vi "Periodic Tasks.vi"(8 "error in":errorcluster) -> ()   [LabVIEW 2020]
doc: "This VI runs in parallel to other tasks. It can contain as many user-defined periodic loops as you need. These can carry out PID or other sorts of timed response."
uses:
  <vilib>/Rock Robotics/WPI/Solenoid/WPI_SolenoidValue.ctl
  <vilib>/Rock Robotics/WPI/Utilities/WPI_GetSetVariantRefNum.vi
  <vilib>/Rock Robotics/Network Tables/NT Write Boolean.vi
  <vilib>/functionblocks/Edge Detection/One Shot Rising with Input/One Shot Rising with Input.vi
  <vilib>/Rock Robotics/Network Tables/NT Write Number.vi
  <vilib>/functionblocks/FB Core/FB Core.xnode
  <vilib>/Rock Robotics/WPI/Solenoid/WPI_SolenoidSetEnum.vi
  <vilib>/functionblocks/NI_FunctionBlock Libraries.lvlib
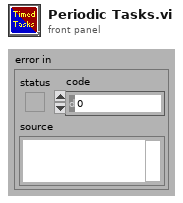
[diagram p1: front panel]
types:
  T1 = enum16{"Wait", "2 Ball", "Button Extend", "Button Retract"}
  T2 = typedef "WPI_JoystickDevRef.ctl" = cluster{"Device":T3}
  T3 = typedef "WPI_JoystickDeviceEnum.ctl" = enum16{"USB 0", "USB 1", "USB 2", "USB 3", "USB 4", "USB 5"}
  T4 = typedef "WPI_RobotDriveDevRef.ctl" = cluster{"DevStatus":errorcluster, "Motors[]":T5[], "Square Inputs":bool, "Max Output":dbl}
  T5 = typedef "WPI_MotorControlDeviceRef.ctl" = cluster{"DeviceStatus":errorcluster, "Type":T6, "PWM":cluster{"PWM Channel":T7, "DeadBand":T8}, "CAN":cluster{"Device Number":u8, "SetOutput VI Ref":variant, "GetOutput VI Ref":variant, "Enable VI Ref":variant, "Disable VI Ref":variant, "Data":variant}, "Invert":bool, "DIO PWM":cluster{"PWM \"Enable\" Channel":T7, "DIOChannel":T9, "PWM Rate":dbl}}
  T6 = typedef "WPI_MotorControlType.ctl" = enum16{"PWM", "CAN", "DIO PWM"}
  T7 = typedef "FPGA_DIOPWMChannel.ctl" = enum8{"PWM 0", "PWM 1", "PWM 2", "PWM 3", "PWM 4", "PWM 5", "PWM 6", "PWM 7", "PWM 8", "PWM 9", "PWM MXP 0", "PWM MXP 1", "PWM MXP 2", "PWM MXP 3", "PWM MXP 4", "PWM MXP 5", "PWM MXP 6", "PWM MXP 7", "PWM MXP 8", "PWM MXP 9", "Invalid"}
  T8 = typedef "WPI_PWMDeadband.ctl" = cluster{"Name":string, "maxPositivePwm":i32, "minPositivePwm":i32, "centerPwm":i32, "maxNegativePwm":i32, "minNegativePwm":i32, "angularRange":u16}
  T9 = typedef "FPGA_DIOChannel.ctl" = enum8{"DIO 0", "DIO 1", "DIO 2", "DIO 3", "DIO 4", "DIO 5", "DIO 6", "DIO 7", "DIO 8", "DIO 9", "DIO MXP 0", "DIO MXP 1", "DIO MXP 2", "DIO MXP 3", "DIO MXP 4", "DIO MXP 5", "DIO MXP 6", "DIO MXP 7", "DIO MXP 8", "DIO MXP 9", "DIO MXP 10", "DIO MXP 11", "DIO MXP 12", "DIO MXP 13", "DIO MXP 14", "DIO MXP 15", "SPI Port CS1", "SPI Port CS2", "SPI Port CS3", "SPI Port MISO", "SPI Port MOSI", "Invalid"}
  T10 = cluster{"JoystickDevRef":T2, "RobotDriveDevRef":T4}
  T11 = typedef "WPI_SolenoidDevRef.ctl" = cluster{"DevStatus":errorcluster, "Pneumatics Control Module":u8, "Forward Solenoid Channel":T12, "Reverse Solenoid Channel":T12}
  T12 = typedef "WPI_SolenoidChannel.ctl" = enum8{"Solenoid 0", "Solenoid 1", "Solenoid 2", "Solenoid 3", "Solenoid 4", "Solenoid 5", "Solenoid 6", "Solenoid 7", "Solenoid 8", "Solenoid 9", "Solenoid 10", "Solenoid 11", "Solenoid 12", "Solenoid 13", "Solenoid 14", "Solenoid 15", "Invalid"}
  T13 = typedef "WPI_DigitalInputDevRef.ctl" = cluster{"DevStatus":errorcluster, "DIO Channel":T9}
  T14 = typedef "WPI_SolenoidValue.ctl" = enum16{"Off", "On", "Forward", "Reverse"}
  T15 = cluster{"Buttons[0]":bool, "Buttons[1]":bool, "Buttons[2]":bool, "Buttons[3]":bool, "Buttons[4]":bool, "Buttons[5]":bool, "Buttons[6]":bool, "Buttons[7]":bool, "Buttons[8]":bool, "Buttons[9]":bool}
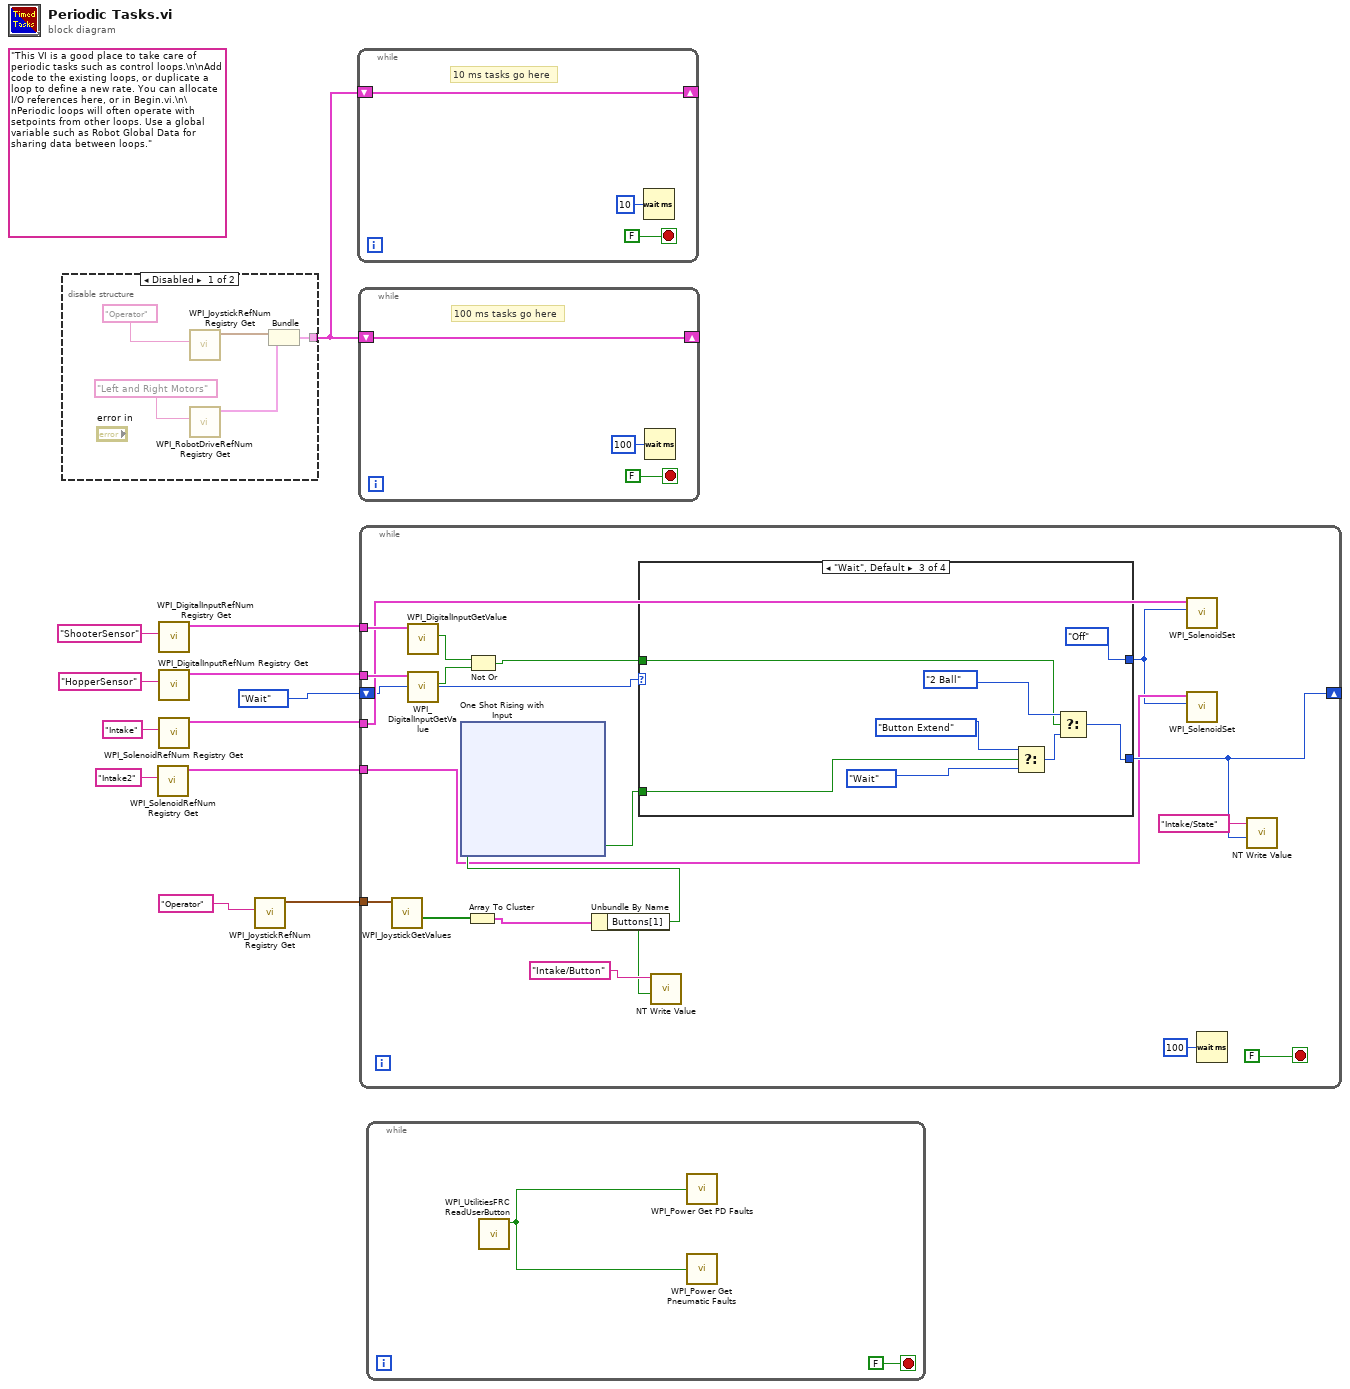
[diagram p0: block diagram]
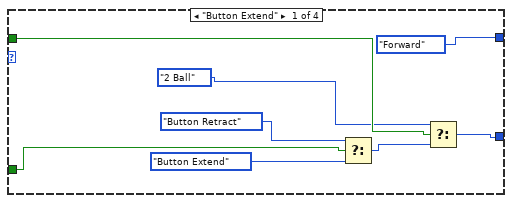
[diagram p2: hidden frame]
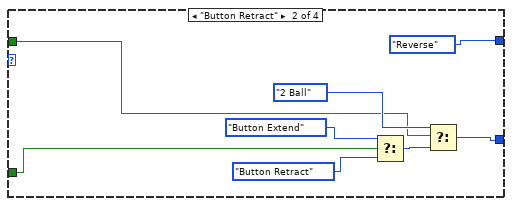
[diagram p3: hidden frame]
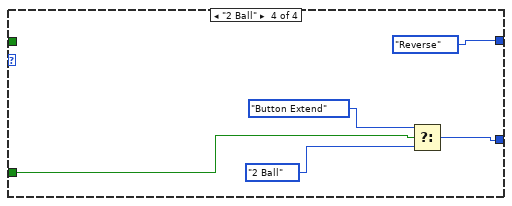
[diagram p4: hidden frame]
diagram:
  (unwired) "This VI is a good place to take care of periodic tasks such as control loops.\n\nAdd code to the existing loops, or duplicate a loop to define a new rate. You can allocate I/O references here, or in Begin.vi.\n\nPeriodic loops will often operate with setpoints from other loops. Use a global variable such as Robot Global Data for sharing data between loops."
  n1 = disable-structure shown="Disabled" {
    disable-tunnel: [w13 _] -> w12
    frame Disabled {
      n2 = call <vilib>:"WPI_JoystickRefNum Registry Get.vi"("refnum name"="Operator") -> ("JoystickDevRef"=w15:T2)  [unwired: 1 in, 9 out]
      n3 = call <vilib>:"WPI_RobotDriveRefNum Registry Get.vi"("refnum name"="Left and Right Motors") -> ("RobotDriveDevRef"=w14:T4)  [unwired: 1 in, 9 out]
      n4 = Bundle("JoystickDevRef"=w15, "RobotDriveDevRef"=w14) -> (w13:T10)  [unwired: 1 out]
    }
    frame Enabled {
    }
  }
  n5 = call <vilib>:"WPI_SolenoidRefNum Registry Get.vi"("refnum name"="Intake2") -> ("SolenoidDevRef"=w1:T11)  [unwired: 9 in, 1 out]
  n6 = call <vilib>:"WPI_DigitalInputRefNum Registry Get.vi"("refnum name"="ShooterSensor") -> ("DigitalInputDevRef"=w7:T13)  [unwired: 9 in, 1 out]
  n7 = call <vilib>:"WPI_DigitalInputRefNum Registry Get.vi"("refnum name"="HopperSensor") -> ("DigitalInputDevRef"=w8:T13)  [unwired: 9 in, 1 out]
  n8 = call <vilib>:"WPI_SolenoidRefNum Registry Get.vi"("refnum name"="Intake") -> ("SolenoidDevRef"=w6:T11)  [unwired: 9 in, 1 out]
  n9 = call <vilib>:"WPI_JoystickRefNum Registry Get.vi"("refnum name"="Operator") -> ("JoystickDevRef"=w3:T2)  [unwired: 9 in, 1 out]
  n10 = while {
    shift-right: [w18] -> _
    shift-left: w12 -> [w18]
    stop <- FALSE stop-if-true
    # "10 ms tasks go here"
    n11 = Wait (ms)(milliseconds to wait=u32 10) -> ()  [unwired: 1 out]
  }
  n12 = while {
    shift-right: [w21] -> _
    shift-left: w12 -> [w21]
    stop <- FALSE stop-if-true
    # "100 ms tasks go here"
    n13 = Wait (ms)(milliseconds to wait=u32 100) -> ()  [unwired: 1 out]
  }
  n14 = while {
    tunnel: w8 -> [w39]
    tunnel: w7 -> [w40]
    tunnel: w6 -> [w36]
    shift-right: [w31] -> _
    shift-left: T1."Wait" -> [w34]
    tunnel: w3 -> [w27]
    tunnel: w1 -> [w25]
    stop <- FALSE stop-if-true
    n15 = call <vilib>:"WPI_JoystickGetValues.vi"("JoystickDevRef"=w27) -> ("Buttons"=w29:bool[])  [unwired: 6 in, 4 out]
    n16 = call <vilib>:"WPI_DigitalInputGetValue.vi"("DigitalInputDevRef"=w40) -> ("Value"=w38:bool)  [unwired: 8 in, 2 out]
    n17 = call <vilib>:"WPI_DigitalInputGetValue.vi"("DigitalInputDevRef"=w39) -> ("Value"=w37:bool)  [unwired: 8 in, 2 out]
    n18 = Array To Cluster(array=w29) -> (cluster=w30:T15)
    n19 = Not Or(1:w37, 2:w38) -> (0:w35:bool)
    n20 = Unbundle By Name(w30) -> ("Buttons[1]"=w26:bool)
    n21 = xnode "One Shot Rising with Input"("input"=w26) -> ("output"=w33:bool)  [unwired: 1 in, 1 out]
    n22 = case shown="\"Wait\", Default" w34 {
      tunnel: [WPI_SolenoidValue."Forward" ("Value") WPI_SolenoidValue."Reverse" ("Value") WPI_SolenoidValue."Off" ("Value") WPI_SolenoidValue."Reverse" ("Value")] -> w24
      tunnel: [w88 w93 w103 w109] -> w31
      tunnel: w33 -> [w81 w89 w97 w105]
      tunnel: w35 -> [w86 w90 w98 _]
      frame "Button Extend" {
        n23 = Select(t=T1."Button Retract", s=w81, f=T1."Button Extend") -> (s? t:f=w84:T1)
        n24 = Select(t=T1."2 Ball", s=w86, f=w84) -> (s? t:f=w88:T1)
      }
      frame "Button Retract" {
        n25 = Select(t=T1."Button Extend", s=w89, f=T1."Button Retract") -> (s? t:f=w94:T1)
        n26 = Select(t=T1."2 Ball", s=w90, f=w94) -> (s? t:f=w93:T1)
      }
      frame "Wait", Default {
        n27 = Select(t=T1."Button Extend", s=w97, f=T1."Wait") -> (s? t:f=w104:T1)
        n28 = Select(t=T1."2 Ball", s=w98, f=w104) -> (s? t:f=w103:T1)
      }
      frame "2 Ball" {
        n29 = Select(t=T1."Button Extend", s=w105, f=T1."2 Ball") -> (s? t:f=w109:T1)
      }
    }
    n30 = call-poly <vilib>:"NT Write Value.vi"("Boolean"=w26, "Name"="Intake/Button") -> ()  [unwired: 9 in, 1 out]
    n31 = call-poly <vilib>:"WPI_SolenoidSet.vi"("Value"=w24, "SolenoidDevRef"=w36) -> ()  [unwired: 8 in, 2 out]
    n32 = call-poly <vilib>:"WPI_SolenoidSet.vi"("Value"=w24, "SolenoidDevRef"=w25) -> ()  [unwired: 8 in, 2 out]
    n33 = Wait (ms)(milliseconds to wait=u32 100) -> ()  [unwired: 1 out]
    n34 = call-poly <vilib>:"NT Write Value.vi"("Numeric"=w31, "Name"="Intake/State") -> ()  [unwired: 9 in, 1 out]
  }
  n35 = while {
    stop <- FALSE stop-if-true
    n36 = call <vilib>:"WPI_UtilitiesFRC ReadUserButton.vi"() -> ("User Button"=w110:bool)  [unwired: 10 in, 1 out]
    n37 = call <vilib>:"WPI_Power Get PD Faults.vi"("Clear Sticky Faults"=w110) -> ()  [unwired: 11 in, 4 out]
    n38 = call <vilib>:"WPI_Power Get Pneumatic Faults.vi"("Clear Sticky Faults"=w110) -> ()  [unwired: 9 in, 6 out]
  }
